vi "FGV - Mode.vi"(6 "Action":enum16{"Read", "Write"}(ring), 8 "Error In":errorcluster, 11 "Mode in":enum16{"Sim", "Real"}(ring)) -> (0 "Error Out":errorcluster, 3 "Mode Out":enum16{"Sim", "Real"}(ring))   [LabVIEW 2020]
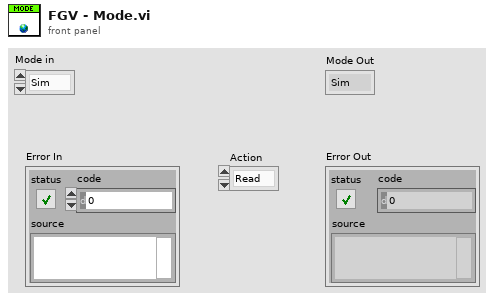
[diagram p1: front panel]
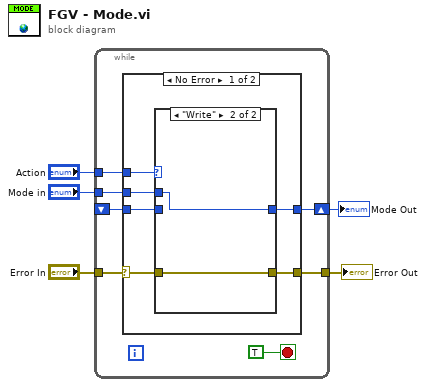
[diagram p0: block diagram]
diagram:
  n1 = while {
    tunnel: "Error In" -> [w12]
    tunnel: [w11] -> w4
    tunnel: "Action" -> [w9]
    tunnel: "Mode in" -> [w8]
    shift-right: [w7] -> w1
    shift-left: _ -> [w6]
    stop <- TRUE stop-if-true
    n2 = case shown="No Error" w12 {
      selector: w12 -> [w18 w24]
      tunnel: [w17 w24] -> w11
      tunnel: w9 -> [w16 _]
      tunnel: w8 -> [w15 _]
      tunnel: [w14 w23] -> w7
      tunnel: w6 -> [w13 w23]
      frame No Error {
        n3 = case shown="\"Write\"" w16 {
          tunnel: w18 -> [w20 w22]
          tunnel: w15 -> [_ w21]
          tunnel: [w20 w22] -> w17
          tunnel: [w19 w21] -> w14
          tunnel: w13 -> [w19 _]
          frame "Read" {
          }
          frame "Write" {
          }
        }
      }
      frame Error {
      }
    }
  }
  "Error Out" <- w4
  "Mode Out" <- w1
